vi "imp_test_v11_p1.vi"() -> ()   [LabVIEW 2014]
uses:
  <vilib>/LabVIEW Targets/FPGA/cRIO/shared/nicrio_ModuleControls/nicrio_cRIO-9237_DataRatesRing.ctl
  <vilib>/LabVIEW Targets/FPGA/cRIO/shared/nicrio_ModuleControls/nicrio_cRIO-9237_ExcitationVoltageRing.ctl
  <vilib>/rvi/FXPMathLib/FxpSinAndCos/subVIs/nifxpmath_SinAndCos_SimConfig.ctl
  <vilib>/rvi/Emulation/niFpgaGetClockAttributes.vi
  <vilib>/rvi/Emulation/niFpgaSctlEmulationGetInTimedLoop.vi
  <vilib>/rvi/Emulation/niFpgaEmulationReportErrorSimple.vi
  <vilib>/rvi/Emulation/niFpgaProcessEmulError.vi
  <vilib>/rvi/interface/RandomDataEmulation/nirviRandomDataMultiElementFPGAFIFO.vi
  <instcachedir>/0/nirviRandomDataMultiElementFPGAFIFO_AD0CFC12EF974623A9C2E4184BC062B2.lvgen/nirviRandomDataMultiElementFPGAFIFO_AD0CFC12EF974623A9C2E4184BC062B2_028.vi
  <vilib>/rvi/interface/RandomDataEmulation/niFpgaRandomDataHandleErrors.vi
  <vilib>/rvi/Emulation/niFpgaCriticalErrorInLSC.vi
  <vilib>/rvi/FXPMathLib/FxpSinAndCos/simVIs/DllFxpSinAndCosTemp_sub.vi
  <vilib>/rvi/eio/common/nirviEmuTemplateMethod_errors.vi
  <vilib>/rvi/eio/common/nirviEmuTemplatePropertySet_errors.vi
  <vilib>/rvi/DataTransferAndStorage/Container/XNode/niFpgaContainer.xnode
  <vilib>/rvi/interface/RandomDataEmulation/nirviRandomDataFpgaMultiElementTemplate.vi
  <vilib>/rvi/Analysis/measure/butterworth/XNode/niFpgaButterworthFilter.xnode
  <vilib>/rvi/FXPMathLib/FxpSinAndCos/XNode/nifxpmath_SinAndCos.xnode
  <vilib>/eio/EIONode/EIONode.xnode
  <vilib>/eio/EIOPropertyNode/EIOPropertyNode.xnode
  <vilib>/rvi/eio/common/nirviEmuTemplatePropertyGet_errors.vi
  <vilib>/rvi/eio/common/nirviEmuTemplatePropertyGet_noerrors.vi
  <vilib>/rvi/eio/common/nirviEmuTemplatePropertySet_noerrors.vi
panel:
  in  "Mavg f loop(uSec)":u32
  in  "F_Threshold_p":fxp<+,12,4>
  out "omega_p (Mavg)":fxp<+/-,36,13>
  out "Dp_d (Mavg)":fxp<+/-,36,13>
  out "omega_p2 (Mavg)":fxp<+/-,36,14>
  out "Dp2_d (Mavg)":fxp<+/-,36,14>
  in  "mt0_p2":u32
  out "Dp_d (Mavg w. f.)":fxp<+/-,36,14>
  in  "Dp_d (Mavg) coeff.":i32[](array[numeric])=[946630756, 63555534]
  out "omega_p (Mavg w. f)":fxp<+/-,36,14>
  in  "omega_P(Mavg) coeff.":i32[](array[numeric])=[946630756, 63555534]
  out "PID (kHz)":fxp<+/-,20,10>
  in  "Set 6":bool
  in  "Set 5":bool
  in  "Set 4":bool
  in  "Set 3":bool
  in  "Set 2":bool
  in  "Set 1":bool
  out "Dp1_d (T)":fxp<+/-,36,13>
  out "omega_p1 (T)":fxp<+/-,36,13>
  out "Dp2_d (T)":fxp<+/-,36,13>
  out "omega_p2 (T)":fxp<+/-,36,13>
  out "mt_omega_p2":u32
  out "Encoder Position_p2":i32
  out "D_p2":fxp<+/-,32,7>
  out "rad_p2":fxp<+/-,33,20>
  out "D_p1":fxp<+/-,32,7>
  out "rad_p1":fxp<+/-,33,20>
  out "Encoder Position_p1":i32
  out "Dp1_d (Mavg)":fxp<+/-,36,14>
  out "omega_p1 (Mavg)":fxp<+/-,36,14>
  in  "Dp_d_M_avg_Tc (uSec)":i32
  out "Dp_d (T)":fxp<+/-,36,13>
  out "omega_p (T)":fxp<+/-,36,13>
  in  "Vp. Est.":i16(ring) items=["T", "Mavg", "Mavg w. f."]
  in  "Mag. factor_p":fxp<+/-,20,3>
  in  "Mag. encoder_p":bool
  in  "Belt_out_p":fxp<+/-,7,7>
  in  "Belt_in_p":fxp<+/-,6,6>
  out "Fp_dc":fxp<+/-,32,10>
  in  "Zero_p":bool
  in  "mt0_p1":u32
  in  "Encoder reset":bool
  out "fpt_d":fxp<+/-,36,18>
  out "Dp_error_dd":fxp<+/-,36,16>
  out "Dp_error_d":fxp<+/-,33,8>
  in  "Dp_dd coeff.":i32[](array[numeric])=[946630756, 63555534]
  out "Dp_dd":fxp<+/-,36,25>
  out "dFp_PID":fxp<+/-,36,18>
  in  "dFp_PID coeff.":i32[](array[numeric])=[946630756, 63555534]
  out "fpt_i":fxp<+/-,34,18>
  in  "Bv_p":fxp<+/-,22,8>
  in  "Kv_p":fxp<+/-,22,8>
  out "Dp_error":fxp<+/-,22,7>
  out "Dpr_sin":fxp<+/-,22,7>
  in  "Sin offset_p":fxp<+/-,22,7>
  in  "Sin magnitude_p":fxp<+/-,21,6>
  out "Dpr_sin_dd":fxp<+/-,35,20>
  out "Dpr_sin_d":fxp<+/-,33,15>
  out "Sin omega_p":fxp<+/-,34,9>
  in  "Sin wave freq._p (Hz)":fxp<+/-,32,6>
  in  "Dpr_step":fxp<+/-,22,7>
  out "Dpr_for":fxp<+/-,22,7>
  in  "Command_p":i16(ring) items=["Step", "Sine"]
  in  "Ki_p":fxp<+/-,30,9>
  out "Fp_PID":fxp<+/-,36,16>
  in  "fp_tolorance":fxp<+,22,6>
  out "fp_tilde":fxp<+/-,33,10>
  in  "Kd_p":fxp<+/-,30,9>
  in  "Kp_p":fxp<+/-,32,13>
  out "Fr_p":fxp<+/-,32,10>
  in  "S/F coeff_p":fxp<+/-,25,-10>
  out "va_p":fxp<+/-,36,7>
  out "vb_p":fxp<+/-,37,8>
  out "vq_p_F":fxp<+/-,20,5> format="%.57g"
  out "vd_p_F":fxp<+/-,20,5>
  in  "dFp_add":bool
  in  "Stop motor_p":bool
  out "Force_p":fxp<+/-,32,10>
  in  "Strain selection_p":i16(ring) items=["Raw", "Avg.8", "Avg.8 w. filter"]
  out "Strain_p (Avg8 w. f)":fxp<+/-,36,8>
  in  "Strain_p Avg.8 coeff.":i32[](array[numeric])=[946630756, 63555534]
  out "Strain_p (Avg8)":fxp<+/-,36,4>
  out "Raw Strain_p":fxp<+/-,36,4>
  out "Mod6/AI3":fxp<+/-,36,4>
  in  "Strain gage reset_p":bool
  out "Dp_d (mm/s)":fxp<+/-,36,13>
  out "omega_p (rad/s)":fxp<+/-,36,13>
  out "mt_omega_p1":u32
  out "rad_p(NrTheta)":fxp<+/-,33,20>
  out "D_p(mm)":fxp<+/-,32,7>
  out "Encoder Position_p":i32
  in  "Encoder reset_p":bool
  out "Time now(s)":fxp<+,52,14>
  in  "Drive mode":i16(ring) items=["Backward", "Forward", "Imp"]
  in  "Ini coe.":bool
  out "Loop rate (kHz)":fxp<+/-,36,7>
  in  "Stop (Strain)":bool
  in  "Excitation Voltage":T1 items=["2.5 Volts", "3.3 Volts", "5.0 Volts", "10.0 Volts", "External Excitation"]
  in  "Data Rate":T2=1 items=["50.000 kS/s (NI 9237)"=1, "25.000 kS/s (NI 9237)"=2, "16.667 kS/s (NI 9237)"=3, "12.500 kS/s (NI 9237)"=4, "10.000 kS/s (NI 9237)"=5, "8.333 kS/s (NI 9237)"=6, "7.143 kS/s (NI 9237)"=7, "6.250 kS/s (NI 9237)"=8, "5.556 kS/s (NI 9237)"=9, "5.000 kS/s (NI 9237)"=10, "4.545 kS/s (NI 9237)"=11, "4.167 kS/s (NI 9237)"=12, "3.846 kS/s (NI 9237)"=13, "3.571 kS/s (NI 9237)"=14, "3.333 kS/s (NI 9237)"=15, "3.125 kS/s (NI 9237)"=16, "2.941 kS/s (NI 9237)"=17, "2.778 kS/s (NI 9237)"=18, "2.632 kS/s (NI 9237)"=19, "2.500 kS/s (NI 9237)"=20, "2.381 kS/s (NI 9237)"=21, "2.273 kS/s (NI 9237)"=22, "2.174 kS/s (NI 9237)"=23, "2.083 kS/s (NI 9237)"=24, "2.000 kS/s (NI 9237)"=25, "1.923 kS/s (NI 9237)"=26, "1.852 kS/s (NI 9237)"=27, "1.786 kS/s (NI 9237)"=28, "1.724 kS/s (NI 9237)"=29, "1.667 kS/s (NI 9237)"=30, "1.613 kS/s (NI 9237)"=31]
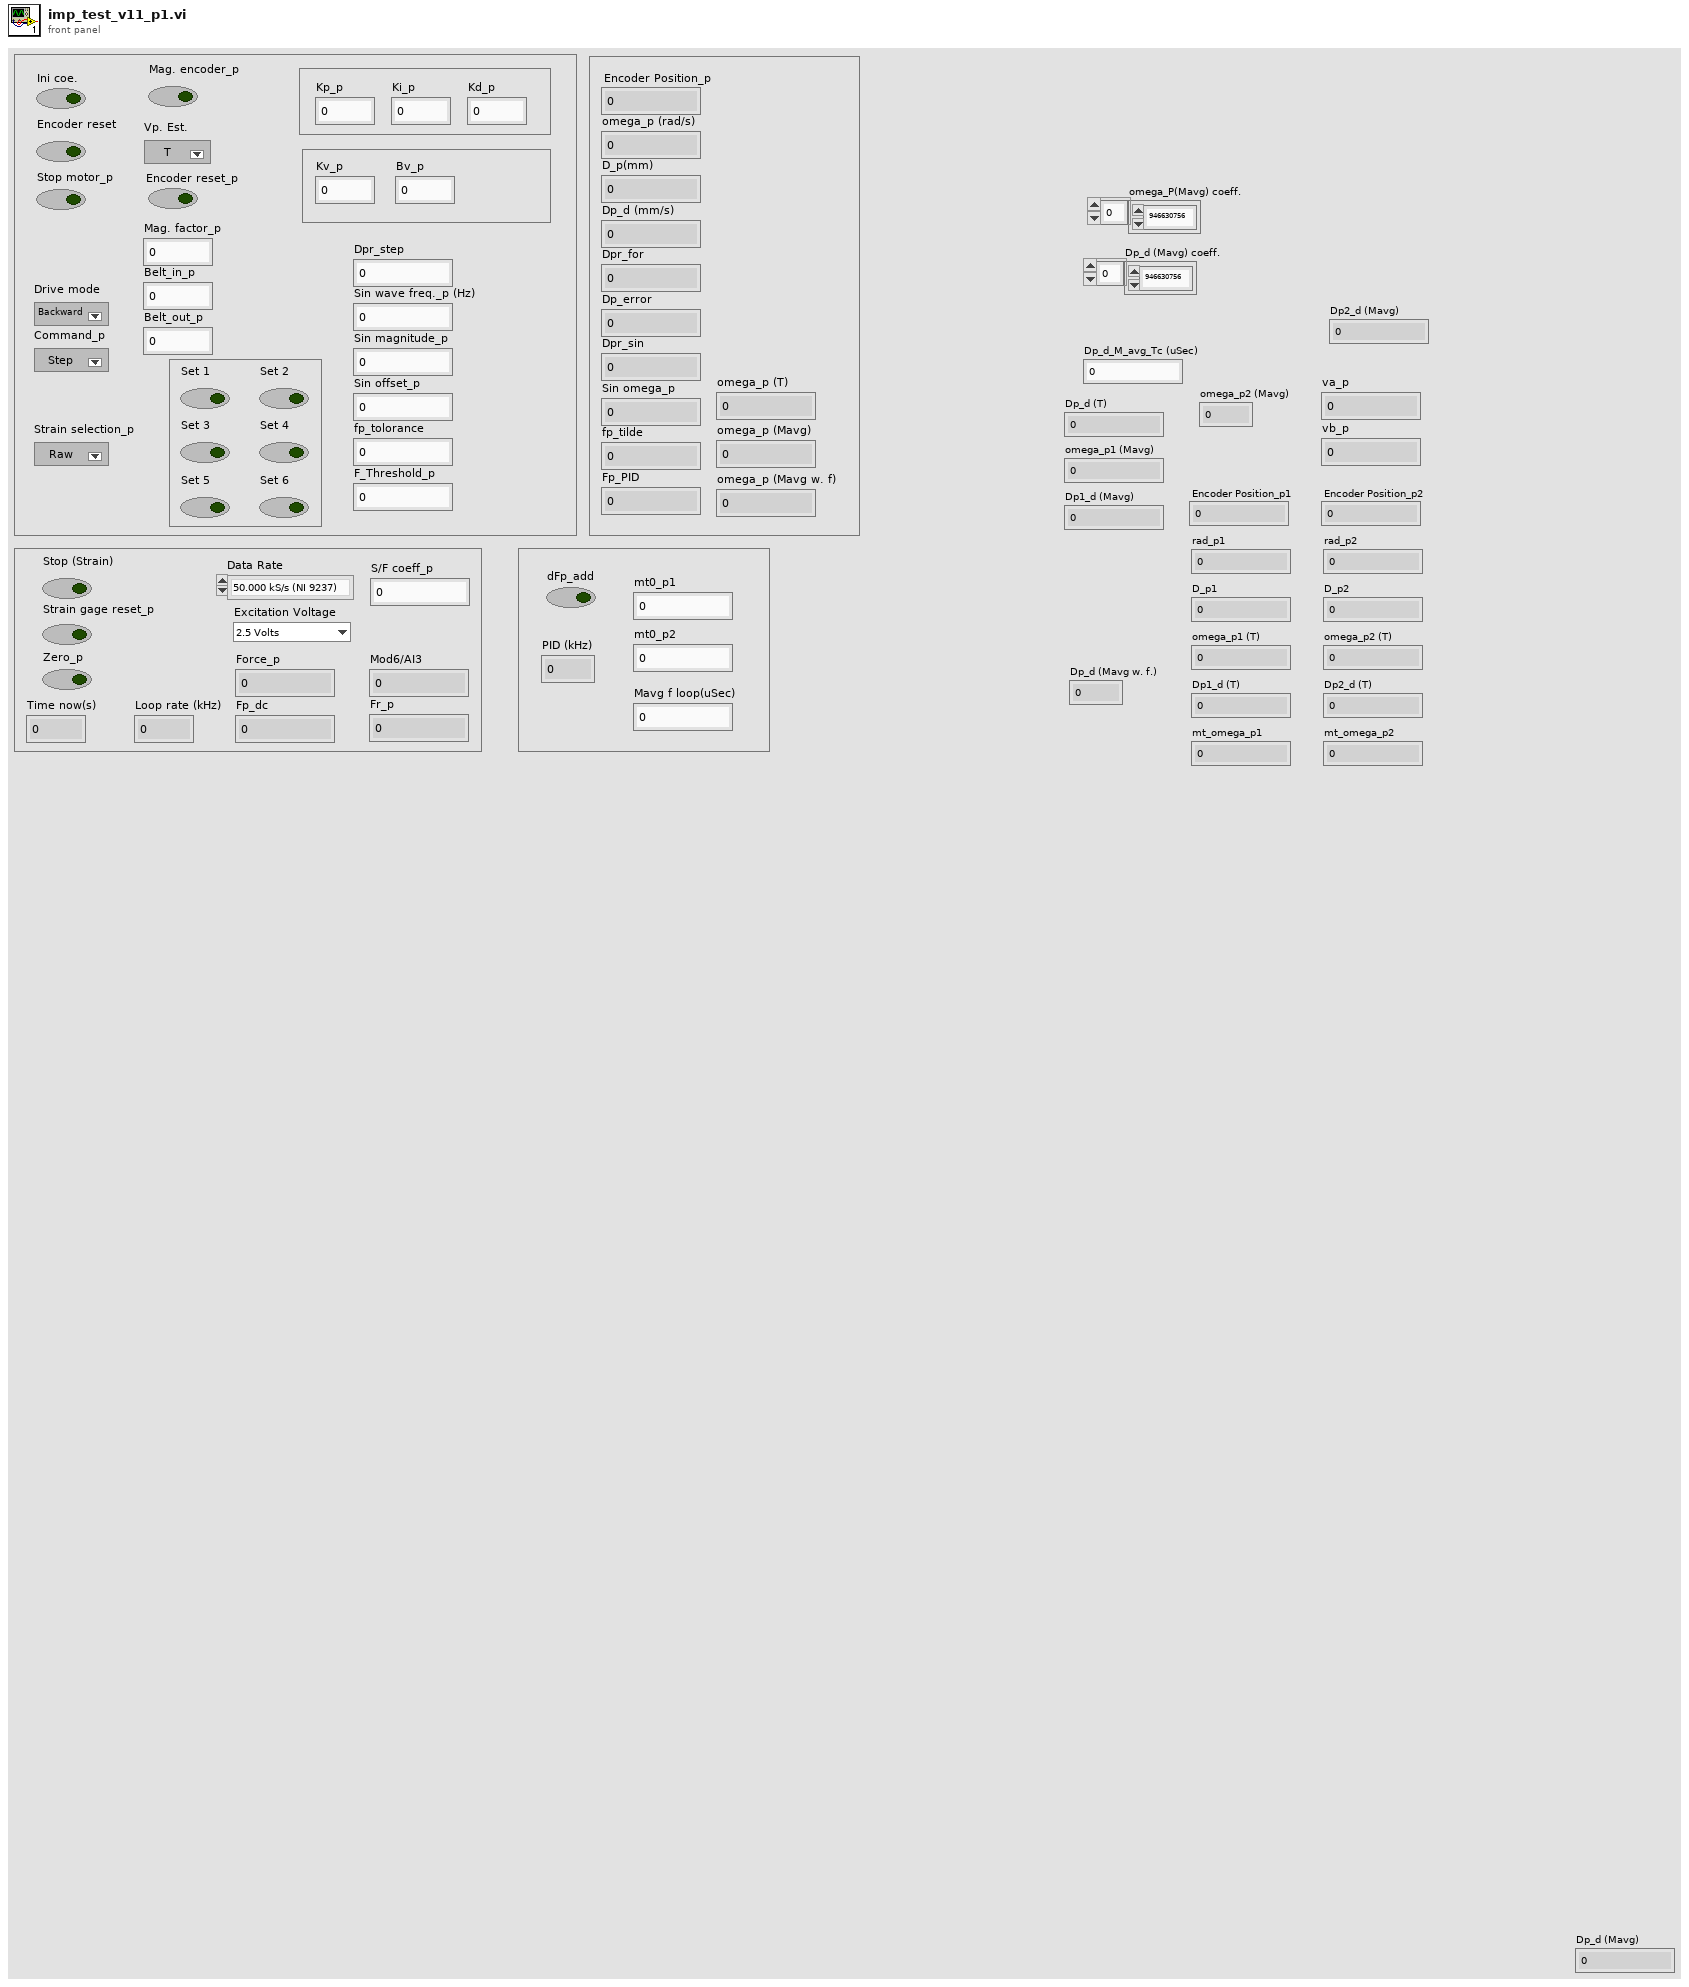
[diagram p1: front panel]
types:
  T1 = typedef "nicrio_cRIO-9237_ExcitationVoltageRing.ctl" = u8
  T2 = typedef "nicrio_cRIO-9237_DataRatesRing.ctl" = u8
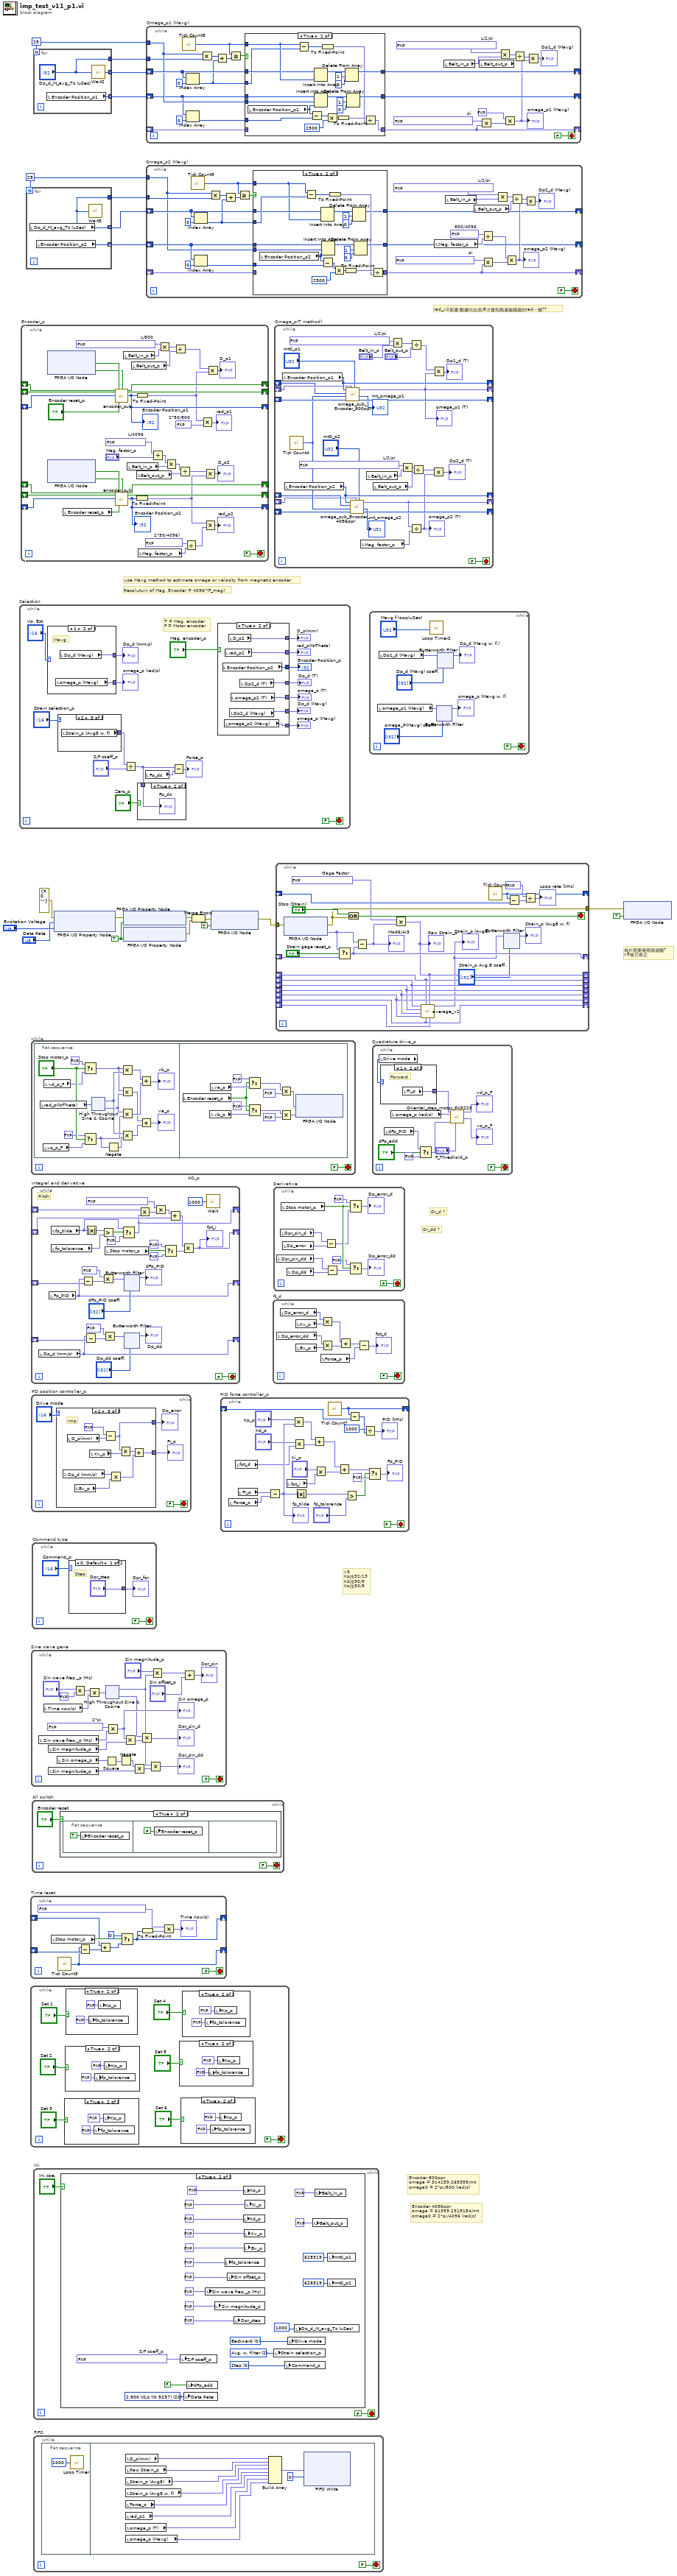
[diagram p0: block diagram]
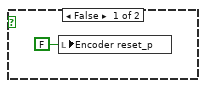
[diagram p10: hidden frame]
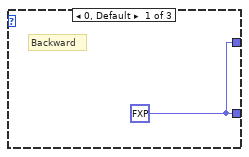
[diagram p11: hidden frame]
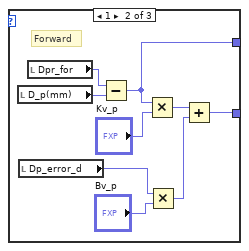
[diagram p12: hidden frame]
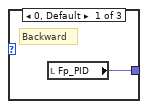
[diagram p13: hidden frame]
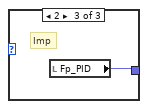
[diagram p14: hidden frame]
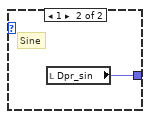
[diagram p15: hidden frame]
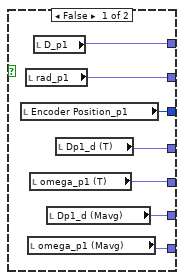
[diagram p16: hidden frame]
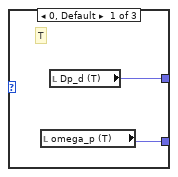
[diagram p17: hidden frame]
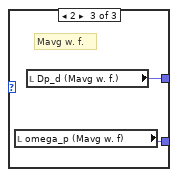
[diagram p18: hidden frame]
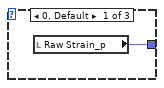
[diagram p20: hidden frame]
diagram:
  w2 = 25
  w8 = 25
  w13 = TRUE ("Half-Bridge Enable")
  # "rad_x2那邊:數據叫出來/8才會和馬達編碼器的rad一樣??"
  # "Encoder 4096ppr\nomega = 61359.2315154/mt\nomega0 = 2*pi/4096 (rad/s)"
  # "Encoder 800ppr\nomega = 314159.265359/mt\nomega0 = 2*pi/800 (rad/s)"
  # "v9\nKp改32/13\nKd改30/9\nKo改30/9"
  # "Resolutuin of Mag. Encoder = 4096*(F_mag)"
  # "use Mavg method to estimate omega or velocity from magnetic encoder"
  # "為什麼要寫兩個迴圈?\nv9後已修正"
  # "Dr_dd ?"
  # "Dr_d ?"
  n1 = while "Selection" {
    stop <- FALSE stop-if-true
    # "T = Mag. encoder\nF = Motor encoder"
    n2 = case shown="1" "Vp. Est." {
      tunnel: [w55 w56 w59] -> w31
      tunnel: [w54 w57 w58] -> w32
      frame 0, Default {
        # "T"
        n3 = local read "omega_p (T)"() -> (w55:fxp<+/-,36,13>)
        n4 = local read "Dp_d (T)"() -> (w54:fxp<+/-,36,13>)
      }
      frame 1 {
        # "Mavg"
        n5 = local read "omega_p (Mavg)"() -> (w56:fxp<+/-,36,13>)
        n6 = local read "Dp_d (Mavg)"() -> (w57:fxp<+/-,36,13>)
      }
      frame 2 {
        # "Mavg w. f."
        n7 = local read "omega_p (Mavg w. f)"() -> (w59:fxp<+/-,36,14>)
        n8 = local read "Dp_d (Mavg w. f.)"() -> (w58:fxp<+/-,36,14>)
      }
    }
    "Dp_d (mm/s)" <- w32
    "omega_p (rad/s)" <- w31
    n9 = case shown="2" "Strain selection_p" {
      tunnel: [w61 w62 w63] -> w38
      frame 0, Default {
        n10 = local read "Raw Strain_p"() -> (w61:fxp<+/-,36,4>)
      }
      frame 1 {
        n11 = local read "Strain_p (Avg8)"() -> (w62:fxp<+/-,36,4>)
      }
      frame 2 {
        n12 = local read "Strain_p (Avg8 w. f)"() -> (w63:fxp<+/-,36,8>)
      }
    }
    n13 = Divide(x=w38, y="S/F coeff_p") -> (x/y=w35:fxp<+/-,32,10>)
    n14 = case shown="True" "Zero_p" {
      tunnel: w35 -> [_ w60]
      frame False {
      }
      frame True {
        "Fp_dc" <- w60
      }
    }
    n15 = local read "Fp_dc"() -> (w33:fxp<+/-,32,10>)
    n16 = Subtract(x=w35, y=w33) -> (x-y=→"Force_p":fxp<+/-,33,11>)
    n17 = case shown="True" "Mag. encoder_p" {
      tunnel: [w46 w53] -> w27
      tunnel: [w45 w52] -> w28
      tunnel: [w44 w51] -> w29
      tunnel: [w42 w50] -> w25
      tunnel: [w43 w49] -> w24
      tunnel: [w41 w47] -> w23
      tunnel: [w40 w48] -> w22
      frame False {
        n18 = local read "Encoder Position_p1"() -> (w44:i32)
        n19 = local read "rad_p1"() -> (w45:fxp<+/-,33,20>)
        n20 = local read "omega_p1 (Mavg)"() -> (w40:fxp<+/-,36,14>)
        n21 = local read "omega_p1 (T)"() -> (w42:fxp<+/-,36,13>)
        n22 = local read "D_p1"() -> (w46:fxp<+/-,32,7>)
        n23 = local read "Dp1_d (Mavg)"() -> (w41:fxp<+/-,36,14>)
        n24 = local read "Dp1_d (T)"() -> (w43:fxp<+/-,36,13>)
      }
      frame True {
        n25 = local read "Encoder Position_p2"() -> (w51:i32)
        n26 = local read "omega_p2 (Mavg)"() -> (w48:fxp<+/-,36,14>)
        n27 = local read "rad_p2"() -> (w52:fxp<+/-,33,20>)
        n28 = local read "D_p2"() -> (w53:fxp<+/-,32,7>)
        n29 = local read "Dp2_d (Mavg)"() -> (w47:fxp<+/-,36,14>)
        n30 = local read "omega_p2 (T)"() -> (w50:fxp<+/-,36,13>)
        n31 = local read "Dp2_d (T)"() -> (w49:fxp<+/-,36,13>)
      }
    }
    "D_p(mm)" <- w27
    "rad_p(NrTheta)" <- w28
    "Encoder Position_p" <- w29
    "Dp_d (T)" <- w24
    "omega_p (T)" <- w25
    "Dp_d (Mavg)" <- w23
    "omega_p (Mavg)" <- w22
  }
  n32 = while "Encoder_p" {
    shift-right: [w101] -> _
    shift-left: _ -> [w100]
    shift-right: [w102] -> _
    shift-left: _ -> [w99]
    shift-right: [w96] -> _
    shift-left: _ -> [w98]
    shift-right: [w87] -> _
    shift-left: _ -> [w86]
    shift-right: [w88] -> _
    shift-left: _ -> [w89]
    shift-right: [w83] -> _
    shift-left: _ -> [w84]
    stop <- FALSE stop-if-true
    w79 = fxp<+/-,20,-5> 0.00048828125  # L/4096
    w77 = fxp<+/-,16,1> 0.0244140625  # 2*50/4096)
    w95 = fxp<+/-,20,-5> 0.002499997615814209  # L/800
    w69 = fxp<+/-,16,1> 0.125  # 2*50/800
    n33 = xnode "FPGA I/O Node"() -> ("Mod7/DIO0"=w104:bool, "Mod7/DIO1"=w103:bool)  [unwired: 2 in, 2 out]
    n34 = xnode "FPGA I/O Node"() -> ("Mod7/DIO4"=w91:bool, "Mod7/DIO5"=w90:bool)  [unwired: 2 in, 2 out]
    n35 = local read "Encoder reset_p"() -> (w85:bool)
    n36 = call "encoder_sub.vi"("A_pre"=w100, "B_pre"=w99, "Encoder Position_pre"=w98, "A input"=w104, "Encoder Position Reset"="Encoder reset_p", "B input"=w103) -> ("A"=w101:bool, "B"=w102:bool, "Encoder Position (Counts)"=w96:i32)  [unwired: 19 in]
    "Encoder Position_p1" <- w96
    n37 = call "encoder_sub.vi"("A_pre"=w86, "B_pre"=w89, "Encoder Position_pre"=w84, "A input"=w91, "Encoder Position Reset"=w85, "B input"=w90) -> ("A"=w87:bool, "B"=w88:bool, "Encoder Position (Counts)"=w83:i32)  [unwired: 19 in]
    "Encoder Position_p2" <- w83
    n38 = local read "Belt_in_p"() -> (w94:fxp<+/-,6,6>)
    n39 = local read "Belt_in_p"() -> (w80:fxp<+/-,6,6>)
    n40 = local read "Belt_out_p"() -> (w92:fxp<+/-,7,7>)
    n41 = To Fixed-Point(number=w83) -> (fixed-point=w65:fxp<+/-,32,32>)  [unwired: 1 in]
    n42 = To Fixed-Point(number=w96) -> (fixed-point=w70:fxp<+/-,32,32>)  [unwired: 1 in]
    n43 = local read "Belt_out_p"() -> (w82:fxp<+/-,7,7>)
    n44 = local read "Mag. factor_p"() -> (w76:fxp<+/-,20,3>)
    n45 = Divide(x=w79, y="Mag. factor_p") -> (x/y=w78:fxp<+/-,41,13>)
    n46 = Multiply(x=w95, y=w94) -> (x*y=w93:fxp<+/-,26,1>)
    n47 = Multiply(x=w78, y=w80) -> (x*y=w81:fxp<+/-,46,18>)
    n48 = Divide(x=w93, y=w92) -> (x/y=w72:fxp<+/-,33,1>)
    n49 = Divide(x=w81, y=w82) -> (x/y=w67:fxp<+/-,53,18>)
    n50 = Divide(x=w77, y=w76) -> (x/y=w64:fxp<+/-,37,5>)
    n51 = Multiply(x=w70, y=w69) -> (x*y=→"rad_p1":fxp<+/-,33,20>)
    n52 = Multiply(x=w67, y=w65) -> (x*y=→"D_p2":fxp<+/-,37,7>)
    n53 = Multiply(x=w65, y=w64) -> (x*y=→"rad_p2":fxp<+/-,46,16>)
    n54 = Multiply(x=w72, y=w70) -> (x*y=→"D_p1":fxp<+/-,32,7>)
  }
  n55 = for {
    N: w2 -> [_]
    tunnel: [w106] -> w4 mode=indexing
    tunnel: [w105] -> w3 mode=indexing
    tunnel: [w105] -> w1
    n56 = local read "Dp_d_M_avg_Tc (uSec)"() -> (w105:i32)
    n57 = local read "Encoder Position_p2"() -> (w106:i32)
    n58 = call "Wait5"("Count(uSec)"=w105) -> ()  [unwired: 1 out]
  }
  n59 = while "Time reset" {
    shift-right: [w116] -> _
    shift-left: _ -> [w117]
    shift-right: [w111] -> _
    shift-left: _ -> [w112]
    stop <- FALSE stop-if-true
    n60 = local read "Stop motor_p"() -> (w118:bool)
    n61 = call "Tick Count3"() -> ("Tick Count(uSec)"=w116:u32)
    n62 = Subtract(x=w116, y=w117) -> (x-y=w115:u32)
    n63 = Add(x=w112, y=w115) -> (x+y=w114:u32)
    n64 = Select(t=u32 0, s=w118, f=w114) -> (s? t:f=w111:u32)
    n65 = To Fixed-Point(number=w111) -> (fixed-point=w110:fxp<+,32,32>)  [unwired: 1 in]
    n66 = Multiply(x=fxp<+,20,-18> 1.0000003385357559e-06, y=w110) -> (x*y=→"Time now(s)":fxp<+,52,14>)
  }
  n67 = while {
    stop <- FALSE stop-if-true
    n68 = case shown="True" "Set 3" {
      frame False {
      }
      frame True {
        n69 = local write "fp_tolorance"(fxp<+,22,6> 3.0 ("fp_tolorance")) -> ()
        n70 = local write "Kp_p"(fxp<+/-,36,9> 100.0 ("Kp_p")) -> ()
      }
    }
    n71 = case shown="True" "Set 2" {
      frame False {
      }
      frame True {
        n72 = local write "fp_tolorance"(fxp<+,22,6> 1.5 ("fp_tolorance")) -> ()
        n73 = local write "Kp_p"(fxp<+/-,36,9> 50.0 ("Kp_p")) -> ()
      }
    }
    n74 = case shown="True" "Set 1" {
      frame False {
      }
      frame True {
        n75 = local write "fp_tolorance"(fxp<+,22,6> 3.0 ("fp_tolorance")) -> ()
        n76 = local write "Kp_p"(fxp<+/-,36,9> 50.0 ("Kp_p")) -> ()
      }
    }
    n77 = case shown="True" "Set 5" {
      frame False {
      }
      frame True {
        n78 = local write "fp_tolorance"(fxp<+,22,6> 3.0 ("fp_tolorance")) -> ()
        n79 = local write "Kp_p"(fxp<+/-,36,9> 150.0 ("Kp_p")) -> ()
      }
    }
    n80 = case shown="True" "Set 6" {
      frame False {
      }
      frame True {
        n81 = local write "fp_tolorance"(fxp<+,22,6> 1.5 ("fp_tolorance")) -> ()
        n82 = local write "Kp_p"(fxp<+/-,36,9> 150.0 ("Kp_p")) -> ()
      }
    }
    n83 = case shown="True" "Set 4" {
      frame False {
      }
      frame True {
        n84 = local write "fp_tolorance"(fxp<+,22,6> 1.5 ("fp_tolorance")) -> ()
        n85 = local write "Kp_p"(fxp<+/-,36,9> 100.0 ("Kp_p")) -> ()
      }
    }
  }
  n86 = while "AO_p" {
    stop <- FALSE stop-if-true
    n87 = flat-sequence {
      frame #0 {
        n88 = local read "rad_p(NrTheta)"() -> (w150:fxp<+/-,33,20>)
        n89 = local read "vq_p_F"() -> (w151:fxp<+/-,20,5>)
        n90 = local read "vd_p_F"() -> (w153:fxp<+/-,20,5>)
        n91 = Select(t=fxp<+/-,20,5> 0.0, s="Stop motor_p", f=w153) -> (s? t:f=w142:fxp<+/-,20,5>)
        n92 = Select(t=fxp<+,1,1> 0.0, s="Stop motor_p", f=w151) -> (s? t:f=w141:fxp<+/-,20,5>)
        n93 = xnode "High Throughput Sine & Cosine"("x (pi)"=w150) -> ("sin(x)"=w144:fxp<+/-,16,2>, "cos(x)"=w143:fxp<+/-,16,2>)
        n94 = Negate(x=w141) -> (-x=w149:fxp<+/-,21,6>)
        n95 = Multiply(x=w142, y=w144) -> (x*y=w148:fxp<+/-,36,7>)
        n96 = Multiply(x=w142, y=w143) -> (x*y=w146:fxp<+/-,36,7>)
        n97 = Multiply(x=w143, y=w141) -> (x*y=w147:fxp<+/-,36,7>)
        n98 = Multiply(x=w144, y=w149) -> (x*y=w145:fxp<+/-,35,6>)
        n99 = Add(x=w148, y=w147) -> (x+y=→"vb_p":fxp<+/-,37,8>)
        n100 = Add(x=w146, y=w145) -> (x+y=→"va_p":fxp<+/-,36,7>)
      }
      frame #1 {
        n101 = local read "Encoder reset_p"() -> (w186:bool)
        n102 = local read "vb_p"() -> (w187:fxp<+/-,37,8>)
        n103 = local read "va_p"() -> (w188:fxp<+/-,36,7>)
        n104 = Select(t=fxp<+,2,2> 3.0, s=w186, f=w188) -> (s? t:f=w194:fxp<+/-,36,7>)
        n105 = Select(t=fxp<+,1,1> 0.0, s=w186, f=w187) -> (s? t:f=w193:fxp<+/-,37,8>)
        n106 = Multiply(x=w194, y=fxp<+/-,1,0> -0.5) -> (x*y=w189:fxp<+/-,36,6>)
        n107 = Multiply(x=w193, y=fxp<+/-,1,0> -0.5) -> (x*y=w190:fxp<+/-,36,6>)
        n108 = xnode "FPGA I/O Node"("Mod8/AO0"=w189, "Mod8/AO1"=w190) -> ()  [unwired: 2 in, 2 out]
      }
    }
  }
  n109 = while "Sine wave gene" {
    stop <- FALSE stop-if-true
    w202 = fxp<+,20,3> 6.2831878662109375  # 2*pi
    n110 = local read "Sin wave freq._p (Hz)"() -> (w198:fxp<+/-,32,6>)
    n111 = local read "Time now(s)"() -> (w216:fxp<+,52,14>)
    n112 = local read "Sin magnitude_p"() -> (w199:fxp<+/-,21,6>)
    n113 = local read "Sin magnitude_p"() -> (w201:fxp<+/-,21,6>)
    n114 = local read "Sin omega_p"() -> (w200:fxp<+/-,34,9>)
    n115 = Multiply(x="Sin wave freq._p (Hz)", y=fxp<+/-,10,3> 2.0) -> (x*y=w220:fxp<+/-,42,9>)
    n116 = Multiply(x=w220, y=w216) -> (x*y=w217:fxp<+/-,41,19>)
    n117 = Square(x=w200) -> (x^2=w212:fxp<+,34,18>)
    n118 = xnode "High Throughput Sine & Cosine"("x (pi)"=w217) -> ("sin(x)"=w203:fxp<+/-,16,2>, "cos(x)"=w208:fxp<+/-,16,2>)
    n119 = Multiply(x=w202, y=w198) -> (x*y=w215:fxp<+/-,34,9>)
    "Sin omega_p" <- w215
    n120 = Negate(x=w212) -> (-x=w211:fxp<+/-,35,19>)
    n121 = Multiply(x=w215, y=w199) -> (x*y=w214:fxp<+/-,33,15>)
    n122 = Multiply(x=w211, y=w201) -> (x*y=w210:fxp<+/-,35,19>)
    n123 = Multiply(x=w208, y=w214) -> (x*y=→"Dpr_sin_d":fxp<+/-,33,15>)
    n124 = Multiply(x=w203, y=w210) -> (x*y=→"Dpr_sin_dd":fxp<+/-,35,20>)
    n125 = Multiply(x="Sin magnitude_p", y=w203) -> (x*y=w206:fxp<+/-,37,8>)
    n126 = Add(x=w206, y="Sin offset_p") -> (x+y=→"Dpr_sin":fxp<+/-,37,8>)
  }
  n127 = while "Integral and derivative" {
    shift-right: [w274] -> _
    shift-left: _ -> [w277]
    shift-right: [w267] -> _
    shift-left: _ -> [w266]
    shift-right: [w261] -> _
    shift-left: _ -> [w260]
    shift-right: [w256] -> _
    shift-left: _ -> [w257]
    stop <- FALSE stop-if-true
    # "Pitch"
    n128 = local read "Dp_d (mm/s)"() -> (w256:fxp<+/-,36,13>)
    n129 = local read "Fp_PID"() -> (w261:fxp<+/-,36,16>)
    n130 = local read "fp_tilde"() -> (w278:fxp<+/-,33,10>)
    n131 = local read "fp_tolorance"() -> (w281:fxp<+,22,6>)
    n132 = Subtract(x=w261, y=w260) -> (x-y=w265:fxp<+/-,37,17>)
    n133 = Subtract(x=w256, y=w257) -> (x-y=w258:fxp<+/-,37,14>)
    n134 = Absolute Value(x=w278) -> (abs(x)=w282:fxp<+,33,10>)
    n135 = Greater?(x=w282, y=w281) -> (0:w280:bool)
    n136 = Multiply(x=fxp<+,7,10> 1000.0, y=w265) -> (x*y=w263:fxp<+/-,32,18>)
    n137 = Multiply(x=fxp<+,7,10> 1000.0, y=w258) -> (x*y=w254:fxp<+/-,36,21>)
    n138 = local read "Stop motor_p"() -> (w269:bool)
    n139 = Select(t=w278, s=w280, f=fxp<+,1,1> 0.0) -> (s? t:f=w274:fxp<+/-,33,10>)
    n140 = xnode "Butterworth Filter"("input data"=w263, "scaled coefficients"="dFp_PID coeff.") -> ("output data"=→"dFp_PID":fxp<+/-,36,22>)  [unwired: 1 in]
    n141 = xnode "Butterworth Filter"("input data"=w254, "scaled coefficients"="Dp_dd coeff.") -> ("output data"=→"Dp_dd":fxp<+/-,36,25>)  [unwired: 1 in]
    n142 = Multiply(x=w277, y=w274) -> (x*y=w276:fxp<+/-,34,12>)
    n143 = Multiply(x=fxp<+/-,30,12> 0.000499725341796875, y=w276) -> (x*y=w273:fxp<+/-,34,10>)
    n144 = Select(t=fxp<+,1,1> 0.0, s=w269, f=fxp<+,1,1> 1.0) -> (s? t:f=w271:fxp<+,1,1>)
    n145 = Add(x=w273, y=w266) -> (x+y=w272:fxp<+/-,36,16>)
    n146 = Multiply(x=w272, y=w271) -> (x*y=w267:fxp<+/-,34,18>)
    "fpt_i" <- w267
    n147 = call "Wait"("Count(uSec)"=u32 1000) -> ()  [unwired: 1 out]
  }
  n148 = while "PD position controller_p" {
    stop <- FALSE stop-if-true
    n149 = case shown="2" "Drive mode" {
      tunnel: [w304 w307 w314] -> w303
      tunnel: [w304 w305 w319] -> w300
      frame 0, Default {
        w304 = fxp<+/-,62,19> 0.0
        # "Backward"
      }
      frame 1 {
        # "Forward"
        n150 = local read "D_p(mm)"() -> (w313:fxp<+/-,32,7>)
        n151 = local read "Dp_error_d"() -> (w306:fxp<+/-,33,8>)
        n152 = local read "Dpr_for"() -> (w312:fxp<+/-,22,7>)
        n153 = Subtract(x=w312, y=w313) -> (x-y=w305:fxp<+/-,33,8>)
        n154 = Multiply(x=w305, y="Kv_p") -> (x*y=w309:fxp<+/-,54,15>)
        n155 = Multiply(x=w306, y="Bv_p") -> (x*y=w308:fxp<+/-,55,16>)
        n156 = Add(x=w309, y=w308) -> (x+y=w307:fxp<+/-,55,16>)
      }
      frame 2 {
        # "Imp"
        n157 = local read "Dp_d (mm/s)"() -> (w317:fxp<+/-,36,13>)
        n158 = local read "D_p(mm)"() -> (w320:fxp<+/-,32,7>)
        n159 = local read "Bv_p"() -> (w316:fxp<+/-,22,8>)
        n160 = local read "Kv_p"() -> (w322:fxp<+/-,22,8>)
        n161 = Subtract(x=fxp<+/-,32,7> 0.0, y=w320) -> (x-y=w319:fxp<+/-,33,8>)
        n162 = Multiply(x=w317, y=w316) -> (x*y=w315:fxp<+/-,58,21>)
        n163 = Multiply(x=w319, y=w322) -> (x*y=w318:fxp<+/-,54,15>)
        n164 = Add(x=w318, y=w315) -> (x+y=w314:fxp<+/-,60,21>)
      }
    }
    "Fr_p" <- w303
    "Dp_error" <- w300
  }
  n165 = while "Command type" {
    stop <- FALSE stop-if-true
    n166 = case shown="0, Default" "Command_p" {
      tunnel: ["Dpr_step" w327] -> w324
      frame 0, Default {
        # "Step"
      }
      frame 1 {
        # "Sine"
        n167 = local read "Dpr_sin"() -> (w327:fxp<+/-,22,7>)
      }
    }
    "Dpr_for" <- w324
  }
  n168 = while "All switch" {
    stop <- FALSE stop-if-true
    n169 = case shown="True" "Encoder reset" {
      frame False {
        n170 = local write "Encoder reset_p"(FALSE ("Encoder reset_p")) -> ()
      }
      frame True {
        n171 = flat-sequence {
          frame #0 {
            n172 = local write "Encoder reset_p"(TRUE ("Encoder reset_p")) -> ()
          }
          frame #1 {
            n173 = local write "Encoder reset_p"(FALSE ("Encoder reset_p")) -> ()
          }
          frame #2 {
          }
        }
      }
    }
  }
  n174 = for {
    N: w8 -> [_]
    tunnel: ["Dp_d_M_avg_Tc (uSec)"] -> w5
    tunnel: [w334] -> w7 mode=indexing
    tunnel: [w333] -> w6 mode=indexing
    n175 = local read "Encoder Position_p1"() -> (w333:i32)
    n176 = call "Wait2"("Count(uSec)"="Dp_d_M_avg_Tc (uSec)") -> ("Tick Count(uSec)"=w334:u32)
  }
  n177 = while "Ini" {
    stop <- FALSE stop-if-true
    n178 = case shown="True" "Ini coe." {
      frame False {
      }
      frame True {
        w340 = T2 20 items=["50.000 kS/s (NI 9237)"=1, "25.000 kS/s (NI 9237)"=2, "16.667 kS/s (NI 9237)"=3, "12.500 kS/s (NI 9237)"=4, "10.000 kS/s (NI 9237)"=5, "8.333 kS/s (NI 9237)"=6, "7.143 kS/s (NI 9237)"=7, "6.250 kS/s (NI 9237)"=8, "5.556 kS/s (NI 9237)"=9, "5.000 kS/s (NI 9237)"=10, "4.545 kS/s (NI 9237)"=11, "4.167 kS/s (NI 9237)"=12, "3.846 kS/s (NI 9237)"=13, "3.571 kS/s (NI 9237)"=14, "3.333 kS/s (NI 9237)"=15, "3.125 kS/s (NI 9237)"=16, "2.941 kS/s (NI 9237)"=17, "2.778 kS/s (NI 9237)"=18, "2.632 kS/s (NI 9237)"=19, "2.500 kS/s (NI 9237)"=20, "2.381 kS/s (NI 9237)"=21, "2.273 kS/s (NI 9237)"=22, "2.174 kS/s (NI 9237)"=23, "2.083 kS/s (NI 9237)"=24, "2.000 kS/s (NI 9237)"=25, "1.923 kS/s (NI 9237)"=26, "1.852 kS/s (NI 9237)"=27, "1.786 kS/s (NI 9237)"=28, "1.724 kS/s (NI 9237)"=29, "1.667 kS/s (NI 9237)"=30, "1.613 kS/s (NI 9237)"=31] ("Data Rate")
        w355 = i16 0 items=["Step", "Sine"] ("Command_p")
        w356 = i16 2 items=["Raw", "Avg.", "Avg. w. filter"] ("Strain selection_p")
        w357 = fxp<+/-,25,-10> 5.851034075021744e-07  # S/F coeff_p
        w358 = i16 0 items=["Backward", "Forward"] ("Drive mode")
        n179 = local write "S/F coeff_p"(w357) -> ()
        n180 = local write "Data Rate"(w340) -> ()
        n181 = local write "dFp_add"(FALSE ("dFp_add")) -> ()
        n182 = local write "Sin wave freq._p (Hz)"(fxp<+/-,32,6> 1.0 ("Sin wave freq._p (Hz)")) -> ()
        n183 = local write "Sin magnitude_p"(fxp<+/-,21,6> 5.0 ("Sin magnitude_p")) -> ()
        n184 = local write "fp_tolorance"(fxp<+,22,6> 5.0 ("fp_tolorance")) -> ()
        n185 = local write "Sin offset_p"(fxp<+/-,22,7> 0.0 ("Sin offset_p")) -> ()
        n186 = local write "Dpr_step"(fxp<+/-,22,7> 0.0 ("Dpr_step")) -> ()
        n187 = local write "Kp_p"(fxp<+/-,36,9> 30.0 ("Kp_p")) -> ()
        n188 = local write "Kd_p"(fxp<+/-,36,9> 0.0 ("Kd_p")) -> ()
        n189 = local write "Kv_p"(fxp<+/-,22,8> 0.0 ("Kv_p")) -> ()
        n190 = local write "Bv_p"(fxp<+/-,22,8> 0.0 ("Bv_p")) -> ()
        n191 = local write "Ki_p"(fxp<+/-,36,9> 0.0 ("Ki_p")) -> ()
        n192 = local write "Strain selection_p"(w356) -> ()
        n193 = local write "Command_p"(w355) -> ()
        n194 = local write "Drive mode"(w358) -> ()
        n195 = local write "Dp_d_M_avg_Tc (uSec)"(u32 1000 ("D_d_M_avg_Tc (uSec)")) -> ()
        n196 = local write "Belt_out_p"(fxp<+/-,7,7> 36.0 ("Belt_op")) -> ()
        n197 = local write "Belt_in_p"(fxp<+/-,6,6> 16.0 ("Belt_mp")) -> ()
        n198 = local write "mt0_p1"(u32 628319 ("mt0_p1")) -> ()
        n199 = local write "mt0_p2"(u32 628319 ("mt0_p2")) -> ()
      }
    }
  }
  n200 = while "FIFO" {
    stop <- FALSE stop-if-true
    n201 = flat-sequence {
      frame #0 {
        n202 = call "Loop Timer"("Count(uSec)"=u32 1000) -> ()  [unwired: 1 out]
      }
      frame #1 {
        n203 = local read "D_p(mm)"() -> (w368:fxp<+/-,32,7>)
        n204 = local read "Raw Strain_p"() -> (w367:fxp<+/-,36,4>)
        n205 = local read "Strain_p (Avg8)"() -> (w366:fxp<+/-,36,4>)
        n206 = local read "Strain_p (Avg8 w. f)"() -> (w365:fxp<+/-,36,8>)
        n207 = local read "Force_p"() -> (w364:fxp<+/-,32,10>)
        n208 = local read "rad_p1"() -> (w363:fxp<+/-,33,20>)
        n209 = local read "omega_p (T)"() -> (w362:fxp<+/-,36,13>)
        n210 = local read "omega_p (Mavg)"() -> (w361:fxp<+/-,36,13>)
        n211 = Build Array(w368, w367, w366, w365, w364, w363, w362, w361) -> (w369:fxp<+/-,52,20>[])
        n212 = xnode ("FIFO Write")("Element"=w369, "Timeout"=0) -> ()  [unwired: 1 in, 2 out]
      }
    }
  }
  n213 = xnode "FPGA I/O Property Node"("error in"=errorcluster {"status"=FALSE, "code"=0, "source"=""}, "Data Rate"="Data Rate", "Excitation Voltage"="Excitation Voltage") -> ("error out"=w18:errorcluster)  [unwired: 1 in, 1 out]
  n214 = xnode "FPGA I/O Property Node"("error in"=w18, "Half-Bridge Enable"=w13) -> ("error out"=w11:errorcluster)  [unwired: 1 in, 1 out]
  n215 = xnode "FPGA I/O Property Node"("Half-Bridge Enable"=w13) -> ("error out"=w10:errorcluster)  [unwired: 2 in, 1 out]
  n216 = while "Omega_p2 (Mavg)" {
    shift-right: [w372] -> _
    shift-left: w4 -> [w393]
    shift-right: [w373] -> _
    shift-left: w3 -> [w391]
    shift-right: [w377] -> _
    shift-left: _ -> [w375]
    tunnel: w2 -> [w389]
    tunnel: w1 -> [w394]
    stop <- FALSE stop-if-true
    w378 = fxp<+/-,27,3> 3.1415926814079285  # pi
    w381 = fxp<+,32,0> 0.1953125  # 800/4096
    w386 = fxp<+/-,32,0> 0.3183098859153688  # L/2/pi
    n217 = call "Tick Count9"() -> ("Tick Count(uSec)"=w388:u32)
    n218 = Index Array(array=w391, index=0) -> (element=w390:i32)
    n219 = Index Array(array=w393, index=0) -> (element=w392:i32)
    n220 = Multiply(x=w389, y=w394) -> (x*y=w397:i32)
    n221 = Add(x=w397, y=w390) -> (x+y=w396:i32)
    n222 = Greater Or Equal?(x=w388, y=w396) -> (x >= y?=w395:bool)
    n223 = case shown="True" w395 {
      tunnel: w393 -> [w401 w416]
      tunnel: w392 -> [_ w408]
      tunnel: w391 -> [w402 w417]
      tunnel: w390 -> [_ w418]
      tunnel: w389 -> [_ w415]
      tunnel: w388 -> [_ w403]
      tunnel: [w401 w406] -> w372
      tunnel: [w402 w405] -> w373
      tunnel: [w400 w404] -> w377
      tunnel: w375 -> [w400 _]
      frame False {
      }
      frame True {
        n224 = local read "Encoder Position_p2"() -> (w407:i32)
        n225 = Subtract(x=w403, y=w418) -> (x-y=w419:u32)
        n226 = Insert Into Array(array=w417, new element=w403) -> (w421:i32[])  [unwired: 1 in]
        n227 = Subtract(x=w407, y=w408) -> (x-y=w412:i32)
        n228 = Insert Into Array(array=w416, index=w415, new element=w407) -> (w422:i32[])
        n229 = To Fixed-Point(number=w419) -> (fixed-point=w409:fxp<+,32,32>)  [unwired: 1 in]
        n230 = Multiply(x=w412, y=2500) -> (x*y=w413:i32)
        n231 = To Fixed-Point(number=w413) -> (fixed-point=w414:fxp<+/-,32,32>)  [unwired: 1 in]
        n232 = Delete From Array(array=w421, length=1, index=0) -> (array with subset deleted=w405:i32[])  [unwired: 1 out]
        n233 = Delete From Array(array=w422, length=1, index=0) -> (array with subset deleted=w406:i32[])  [unwired: 1 out]
        n234 = Divide(x=w414, y=w409) -> (x/y=w404:fxp<+/-,64,32>)
      }
    }
    n235 = local read "Mag. factor_p"() -> (w380:fxp<+/-,20,3>)
    n236 = local read "Belt_in_p"() -> (w383:fxp<+/-,6,6>)
    n237 = local read "Belt_out_p"() -> (w382:fxp<+/-,7,7>)
    n238 = Divide(x=w381, y=w380) -> (x/y=w371:fxp<+/-,32,1>)
    n239 = Multiply(x=w378, y=w377) -> (x*y=w379:fxp<+/-,64,35>)
    n240 = Multiply(x=w386, y=w383) -> (x*y=w387:fxp<+/-,38,6>)
    n241 = Multiply(x=w371, y=w379) -> (x*y=w374:fxp<+/-,64,36>)
    "omega_p2 (Mavg)" <- w374
    n242 = Divide(x=w387, y=w382) -> (x/y=w385:fxp<+/-,45,6>)
    n243 = Multiply(x=w385, y=w374) -> (x*y=→"Dp2_d (Mavg)":fxp<+/-,64,41>)
  }
  n244 = while "Omega_p1 (Mavg)" {
    tunnel: w8 -> [w443]
    shift-right: [w441] -> _
    shift-left: w7 -> [w446]
    shift-right: [w440] -> _
    shift-left: w6 -> [w442]
    shift-right: [w439] -> _
    shift-left: _ -> [w438]
    tunnel: w5 -> [w436]
    stop <- FALSE stop-if-true
    w430 = fxp<+/-,27,3> 3.1415926814079285  # pi
    w429 = fxp<+/-,32,0> 0.3183098859153688  # L/2/pi
    n245 = call "Tick Count5"() -> ("Tick Count(uSec)"=w447:u32)
    n246 = Index Array(array=w446, index=0) -> (element=w445:u32)
    n247 = Index Array(array=w442, index=0) -> (element=w444:i32)
    n248 = Multiply(x=w443, y=w436) -> (x*y=w449:i32)
    n249 = Add(x=w449, y=w445) -> (x+y=w448:u32)
    n250 = Greater Or Equal?(x=w447, y=w448) -> (x >= y?=w437:bool)
    n251 = case shown="True" w437 {
      tunnel: w447 -> [_ w470]
      tunnel: w443 -> [_ w467]
      tunnel: w446 -> [w454 w469]
      tunnel: w445 -> [_ w468]
      tunnel: w444 -> [_ w464]
      tunnel: w442 -> [w453 w466]
      tunnel: [w452 w462] -> w439
      tunnel: [w454 w461] -> w441
      tunnel: [w453 w460] -> w440
      tunnel: w438 -> [w452 _]
      frame False {
      }
      frame True {
        n252 = local read "Encoder Position_p1"() -> (w463:i32)
        n253 = Subtract(x=w470, y=w468) -> (x-y=w471:u32)
        n254 = Subtract(x=w463, y=w464) -> (x-y=w456:i32)
        n255 = Insert Into Array(array=w469, new element=w470) -> (w473:u32[])  [unwired: 1 in]
        n256 = Insert Into Array(array=w466, index=w467, new element=w463) -> (w474:i32[])
        n257 = To Fixed-Point(number=w471) -> (fixed-point=w458:fxp<+,32,32>)  [unwired: 1 in]
        n258 = Multiply(x=w456, y=2500) -> (x*y=w457:i32)
        n259 = To Fixed-Point(number=w457) -> (fixed-point=w465:fxp<+/-,32,32>)  [unwired: 1 in]
        n260 = Delete From Array(array=w473, length=1, index=0) -> (array with subset deleted=w461:u32[])  [unwired: 1 out]
        n261 = Delete From Array(array=w474, length=1, index=0) -> (array with subset deleted=w460:i32[])  [unwired: 1 out]
        n262 = Divide(x=w465, y=w458) -> (x/y=w462:fxp<+/-,64,32>)
      }
    }
    n263 = local read "Belt_in_p"() -> (w434:fxp<+/-,6,6>)
    n264 = local read "Belt_out_p"() -> (w433:fxp<+/-,7,7>)
    n265 = Multiply(x=w430, y=w439) -> (x*y=w435:fxp<+/-,64,35>)
    n266 = Multiply(x=w429, y=w434) -> (x*y=w432:fxp<+/-,38,6>)
    n267 = Multiply(x=fxp<+/-,2,2> 1.0 ("f"), y=w435) -> (x*y=w428:fxp<+/-,64,37>)
    "omega_p1 (Mavg)" <- w428
    n268 = Divide(x=w432, y=w433) -> (x/y=w427:fxp<+/-,45,6>)
    n269 = Multiply(x=w427, y=w428) -> (x*y=→"Dp1_d (Mavg)":fxp<+/-,64,42>)
  }
  n270 = Merge Errors(w11, w10) -> (w12:errorcluster)
  n271 = xnode "FPGA I/O Node"("error in"=w12, "Mod6/Start"=TRUE) -> ("error out"=w16:errorcluster)  [unwired: 1 in, 1 out]
  n272 = while "PID force controller_p" {
    shift-right: [w481] -> _
    shift-left: _ -> [w480]
    stop <- FALSE stop-if-true
    n273 = local read "Force_p"() -> (w493:fxp<+/-,32,10>)
    n274 = local read "fpt_d"() -> (w489:fxp<+/-,36,18>)
    n275 = local read "Fr_p"() -> (w494:fxp<+/-,32,10>)
    n276 = Subtract(x=w494, y=w493) -> (x-y=w491:fxp<+/-,33,11>)
    "fp_tilde" <- w491
    n277 = local read "fpt_i"() -> (w485:fxp<+/-,34,18>)
    n278 = Multiply(x="Kp_p", y=w491) -> (x*y=w487:fxp<+/-,64,23>)
    n279 = Multiply(x="Kd_p", y=w489) -> (x*y=w488:fxp<+/-,64,27>)
    n280 = Absolute Value(x=w491) -> (abs(x)=w500:fxp<+,32,10>)
    n281 = Add(x=w487, y=w488) -> (x+y=w483:fxp<+/-,64,28>)
    n282 = Multiply(x="Ki_p", y=w485) -> (x*y=w484:fxp<+/-,64,27>)
    n283 = call "Tick Count7"() -> ("Tick Count(uSec)"=w481:u32)
    n284 = Add(x=w483, y=w484) -> (x+y=w482:fxp<+/-,64,29>)
    n285 = Greater?(x=w500, y="fp_tolorance") -> (0:w497:bool)
    n286 = Subtract(x=w481, y=w480) -> (x-y=w479:u32)
    n287 = Divide(x=u32 1000, y=w479) -> (x/y=→"PID (kHz)":fxp<+/-,20,7>)
    n288 = Select(t=w482, s=w497, f=fxp<+,1,1> 0.0) -> (s? t:f=→"Fp_PID":fxp<+/-,64,29>)
  }
  n289 = while "ft_d" {
    stop <- FALSE stop-if-true
    n290 = local read "Dp_error_dd"() -> (w507:fxp<+/-,36,16>)
    n291 = local read "Dp_error_d"() -> (w509:fxp<+/-,33,8>)
    n292 = local read "Kv_p"() -> (w510:fxp<+/-,22,8>)
    n293 = local read "Bv_p"() -> (w508:fxp<+/-,22,8>)
    n294 = Multiply(x=w509, y=w510) -> (x*y=w505:fxp<+/-,55,16>)
    n295 = Multiply(x=w507, y=w508) -> (x*y=w506:fxp<+/-,58,24>)
    n296 = local read "Force_p"() -> (w503:fxp<+/-,32,10>)
    n297 = Add(x=w505, y=w506) -> (x+y=w504:fxp<+/-,63,24>)
    n298 = Subtract(x=w504, y=w503) -> (x-y=→"fpt_d":fxp<+/-,63,24>)
  }
  n299 = while "Derivative" {
    stop <- FALSE stop-if-true
    n300 = local read "Dpr_sin_dd"() -> (w519:fxp<+/-,35,20>)
    n301 = local read "Dpr_sin_d"() -> (w521:fxp<+/-,33,15>)
    n302 = local read "Stop motor_p"() -> (w517:bool)
    n303 = local read "Dp_error"() -> (w522:fxp<+/-,22,7>)
    n304 = local read "Dp_dd"() -> (w520:fxp<+/-,36,25>)
    n305 = Subtract(x=w521, y=w522) -> (x-y=w514:fxp<+/-,34,16>)
    n306 = Subtract(x=w519, y=w520) -> (x-y=w518:fxp<+/-,41,26>)
    n307 = Select(t=fxp<+,1,1> 0.0, s=w517, f=w514) -> (s? t:f=→"Dp_error_d":fxp<+/-,34,16>)
    n308 = Select(t=fxp<+/-,41,26> 0.0, s=w517, f=w518) -> (s? t:f=→"Dp_error_dd":fxp<+/-,41,26>)
  }
  n309 = while "Omega_p(T method)" {
    shift-right: [w554] -> _
    shift-left: _ -> [w552]
    shift-right: [w535] -> _
    shift-left: _ -> [w553]
    shift-right: [w550] -> _
    shift-left: _ -> [w551]
    shift-right: [w528] -> _
    shift-left: _ -> [w527]
    shift-right: [w523] -> _
    shift-left: _ -> [w525]
    shift-right: [w531] -> _
    shift-left: _ -> [w530]
    stop <- FALSE stop-if-true
    w542 = fxp<+/-,32,0> 0.3183098859153688  # L/2/pi
    w547 = fxp<+/-,32,0> 0.3183098859153688  # L/2/pi
    n310 = local read "Encoder Position_p1"() -> (w554:i32)
    n311 = local read "Encoder Position_p2"() -> (w528:i32)
    n312 = call "Tick Count4"() -> ("Tick Count(Ticks)"=w529:u32)
    n313 = call "omega_sub_Encoder_800ppr.vi"("mt0"="mt0_p1", "omega_pre"=w553, "ticks_m_pre"=w551, "ticks"=w529, "count_pre"=w552, "count"=w554) -> ("ticks_m"=w550:u32, "mt"=→"mt_omega_p1":u32, "omega"=w535:fxp<+/-,36,13>)  [unwired: 3 in]
    "omega_p1 (T)" <- w535
    n314 = call "omega_sub_Encoder_4096ppr.vi"("mt0"="mt0_p2", "omega_pre"=w525, "ticks_m_pre"=w530, "ticks"=w529, "count_pre"=w527, "count"=w528) -> ("ticks_m"=w531:u32, "mt"=→"mt_omega_p2":u32, "omega"=w523:fxp<+/-,36,13>)  [unwired: 3 in]
    n315 = local read "Mag. factor_p"() -> (w543:fxp<+/-,20,3>)
    n316 = local read "Belt_in_p"() -> (w540:fxp<+/-,6,6>)
    n317 = local read "Belt_out_p"() -> (w539:fxp<+/-,7,7>)
    n318 = Multiply(x=w547, y="Belt_in_p") -> (x*y=w545:fxp<+/-,38,6>)
    n319 = Multiply(x=w542, y=w540) -> (x*y=w541:fxp<+/-,38,6>)
    n320 = Divide(x=w545, y="Belt_out_p") -> (x/y=w536:fxp<+/-,20,1>)
    n321 = Divide(x=w523, y=w543) -> (x/y=w524:fxp<+/-,57,31>)
    "omega_p2 (T)" <- w524
    n322 = Divide(x=w541, y=w539) -> (x/y=w534:fxp<+/-,45,6>)
    n323 = Multiply(x=w534, y=w524) -> (x*y=→"Dp2_d (T)":fxp<+/-,36,13>)
    n324 = Multiply(x=w536, y=w535) -> (x*y=→"Dp1_d (T)":fxp<+/-,36,13>)
  }
  n325 = while {
    tunnel: [w555] -> w9
    shift-right: [w579] -> _
    shift-left: _ -> [w580]
    tunnel: w16 -> [w575]
    shift-right: [w571] -> _
    shift-left: _ -> [w572]
    shift-right: [w567] -> _
    shift-left: _ -> [w566]
    shift-right: [w566] -> _
    shift-left: _ -> [w565]
    shift-right: [w565] -> _
    shift-left: _ -> [w564]
    shift-right: [w564] -> _
    shift-left: _ -> [w563]
    shift-right: [w563] -> _
    shift-left: _ -> [w562]
    shift-right: [w562] -> _
    shift-left: _ -> [w561]
    shift-right: [w561] -> _
    shift-left: _ -> [w560]
    stop <- w574 stop-if-true
    w569 = fxp<+,20,2> 2.115001678466797  # Gage Factor
    n326 = xnode "FPGA I/O Node"("error in"=w575) -> ("error out"=w555:errorcluster, "Mod6/AI3"=w570:fxp<+/-,24,-4>)  [unwired: 1 in, 1 out]
    n327 = Select(t=w570, s="Strain gage reset_p", f=w572) -> (s? t:f=w571:fxp<+/-,24,-4>)
    n328 = Or(x="Stop (Strain)", y=w555) -> (x .or. y?=w574:bool)
    n329 = Subtract(x=w570, y=w571) -> (x-y=w568:fxp<+/-,30,-3>)
    "Mod6/AI3" <- w568
    n330 = Multiply(x=w569, y=w568) -> (x*y=w567:fxp<+/-,50,-1>)
    "Raw Strain_p" <- w567
    n331 = call "average_v2.vi"("Numeric 8"=w560, "Numeric"=w567, "Numeric 7"=w561, "Numeric 2"=w566, "Numeric 6"=w562, "Numeric 5"=w563, "Numeric 4"=w564, "Numeric 3"=w565) -> ("Mean (8pt)"=w559:fxp<+/-,32,4>)  [unwired: 1 in, 2 out]
    "Strain_p (Avg8)" <- w559
    n332 = call "Tick Count"() -> ("Tick Count(uSec)"=w579:u32)
    n333 = xnode "Butterworth Filter"("input data"=w559, "scaled coefficients"="Strain_p Avg.8 coeff.") -> ("output data"=→"Strain_p (Avg8 w. f)":fxp<+/-,36,8>)  [unwired: 1 in]
    n334 = Subtract(x=w579, y=w580) -> (x-y=w578:fxp<+/-,32,16>)
    n335 = Divide(x=fxp<+,7,10> 1000.0, y=w578) -> (x/y=→"Loop rate (kHz)":fxp<+/-,40,27>)
  }
  n336 = while {
    stop <- FALSE stop-if-true
    n337 = local read "omega_p1 (Mavg)"() -> (w596:fxp<+/-,36,14>)
    n338 = local read "Dp1_d (Mavg)"() -> (w592:fxp<+/-,36,14>)
    n339 = call "Loop Timer2"("Count(uSec)"="Mavg f loop(uSec)") -> ()  [unwired: 1 out]
    n340 = xnode "Butterworth Filter"("input data"=w596, "scaled coefficients"="omega_P(Mavg) coeff.") -> ("output data"=→"omega_p (Mavg w. f)":fxp<+/-,36,18>)  [unwired: 1 in]
    n341 = xnode "Butterworth Filter"("input data"=w592, "scaled coefficients"="Dp_d (Mavg) coeff.") -> ("output data"=→"Dp_d (Mavg w. f.)":fxp<+/-,36,18>)  [unwired: 1 in]
  }
  n342 = while "Quadrature drive_p" {
    stop <- FALSE stop-if-true
    n343 = local read "Drive mode"() -> (w614:i16)
    n344 = case shown="1" w614 {
      tunnel: [w624 w625 w626] -> w613
      frame 0, Default {
        # "Backward"
        n345 = local read "Fp_PID"() -> (w624:fxp<+/-,36,16>)
      }
      frame 1 {
        # "Forward"
        n346 = local read "Fr_p"() -> (w625:fxp<+/-,32,10>)
      }
      frame 2 {
        # "Imp"
        n347 = local read "Fp_PID"() -> (w626:fxp<+/-,36,16>)
      }
    }
    n348 = local read "dFp_PID"() -> (w617:fxp<+/-,36,18>)
    n349 = local read "omega_p (rad/s)"() -> (w621:fxp<+/-,36,13>)
    n350 = Select(t=w617, s="dFp_add", f=fxp<+,1,1> 0.0) -> (s? t:f=w620:fxp<+/-,36,18>)
    n351 = call "Oriental_step_motor_PKP225.vi"("F_Threshold"="F_Threshold_p", "dFmr"=w620, "omega"=w621, "Fmr"=w613) -> ("vq_F"=→"vq_p_F":fxp<+/-,36,9>, "vd_F"=→"vd_p_F":fxp<+/-,36,9>)  [unwired: 6 in]
  }
  n352 = xnode "FPGA I/O Node"("error in"=w9, "Mod6/Stop"=TRUE) -> ()  [unwired: 1 in, 2 out]
